vi "LoadWiFi.vi"() -> ()   [LabVIEW 2019]
panel:
  in  "OK Button":bool
  in  "Cancel Button":bool
  in  "Path to SDCard":path=path "/Volumes/boot"
  # "Mount SD Card, and then select the path to the boot folder and hit Copy\n\nThen reboot your Pi with the card in it and try Pinging it."
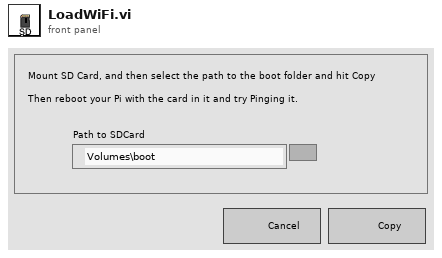
[diagram p1: front panel]
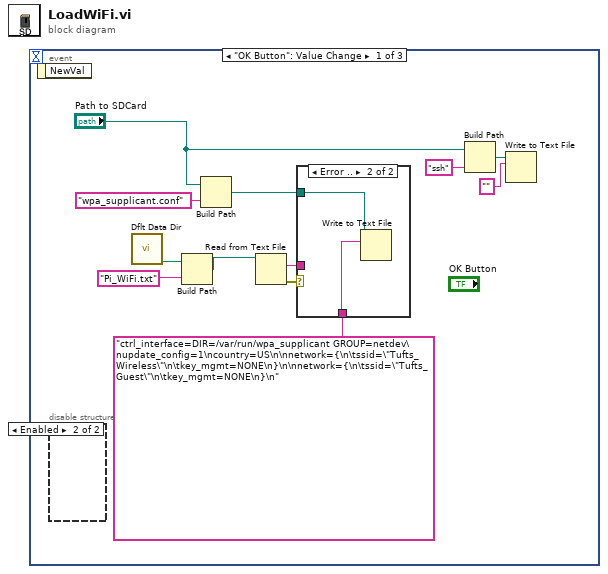
[diagram p0: block diagram]
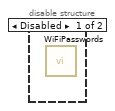
[diagram p2: hidden frame]
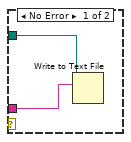
[diagram p3: hidden frame]
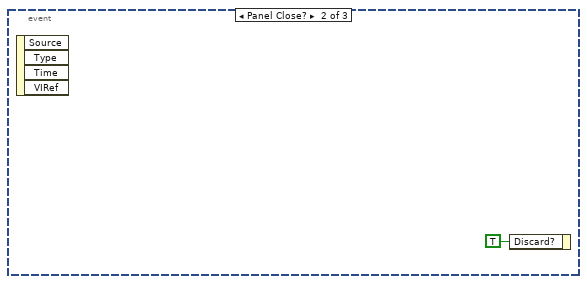
[diagram p4: hidden frame]
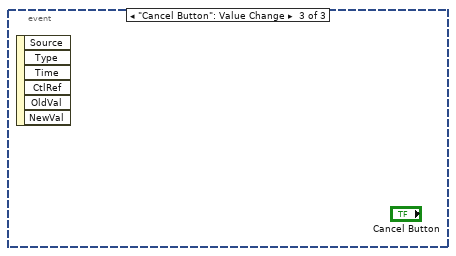
[diagram p5: hidden frame]
diagram:
  n1 = event shown="[0] \"OK Button\": Value Change" {
    selector: _ -> [_ _ _]
    dyn-events: _ -> [_ _ _]
    timeout: _ -> [_ _ _]
    event "OK Button": Value Change {
      n2 = event-data() -> ()  [unwired: 1 in, 1 out]
      n3 = disable-structure shown="Enabled" {
        frame Disabled {
          n4 = call "WiFiPasswords.vi"() -> ()  [unwired: 12 in]
        }
        frame Enabled {
        }
      }
      n5 = call <vilib>:"Dflt Data Dir.vi"() -> ("App:Default Data Directory"=w6:path)
      n6 = Build Path(base path=w6, name or relative path="Pi_WiFi.txt") -> (appended path=w5:path)
      n7 = Build Path(base path="Path to SDCard", name or relative path="wpa_supplicant.conf") -> (appended path=w12:path)
      n8 = Read from Text File(file (use dialog)=w5) -> (text=w3:string, error out=w4:errorcluster)  [unwired: 3 in, 2 out]
      n9 = case shown="Error .." w4 {
        tunnel: w12 -> [w14 w16]
        tunnel: w3 -> [w13 _]
        tunnel: "ctrl_interface=DIR=/var/run/wpa_supplicant GROUP=netdev\nupdate_config=1\ncountry=US\n\nnetwork={\n\tssid=\"Tufts_Wireless\"\n\tkey_mgmt=NONE\n}\n\nnetwork={\n\tssid=\"Tufts_Guest\"\n\tkey_mgmt=NONE\n}\n" ("text") -> [_ w15]
        frame No Error {
          n10 = Write to Text File(file (use dialog)=w14, text=w13) -> ()  [unwired: 2 in, 3 out]
        }
        frame Error {
          n11 = Write to Text File(file (use dialog)=w16, text=w15) -> ()  [unwired: 2 in, 3 out]
        }
      }
      n12 = Build Path(base path="Path to SDCard", name or relative path="ssh") -> (appended path=w10:path)
      n13 = Write to Text File(file (use dialog)=w10, text="") -> ()  [unwired: 2 in, 3 out]
    }
    event Panel Close? {
      n14 = event-data() -> ()  [unwired: 1 in, 4 out]
      n15 = event-data("Discard?"=TRUE) -> ()  [unwired: 1 in, 1 out]
    }
    event "Cancel Button": Value Change {
      n16 = event-data() -> ()  [unwired: 1 in, 6 out]
    }
  }
